vi "仪器参数发送 (子VI).vi"(8 "错误输入":errorcluster caption="错误输出") -> (0 "错误输出":errorcluster)   [LabVIEW 2016, in "数据传输系统.lvlib"]
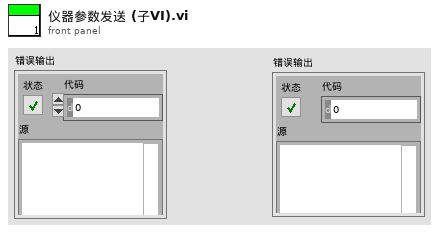
[diagram p1: front panel]
types:
  T1 = cluster{"氨氮仪器参数索引起始时间":string, "总磷仪器参数索引起始时间":string, "总氮仪器参数索引起始时间":string, "CODMn仪器参数索引起始时间":string, "CODCr仪器参数索引起始时间":string, "DO仪器参数索引起始时间":string, "PH仪器参数索引起始时间":string, "比电导率仪器参数索引起始时间":string, "水温仪器参数索引起始时间":string, "浊度仪器参数索引起始时间":string, "叶绿素a仪器参数索引起始时间":string, "藻密度仪器参数索引起始时间":string, "ORP仪器参数索引起始时间":string}
  T2 = cluster{"[0]":string, "[1]":string, "[2]":string, "[3]":string, "[4]":string, "[5]":string, "[6]":string, "[7]":string, "[8]":string, "[9]":string, "[10]":string, "[11]":string, "[12]":string}
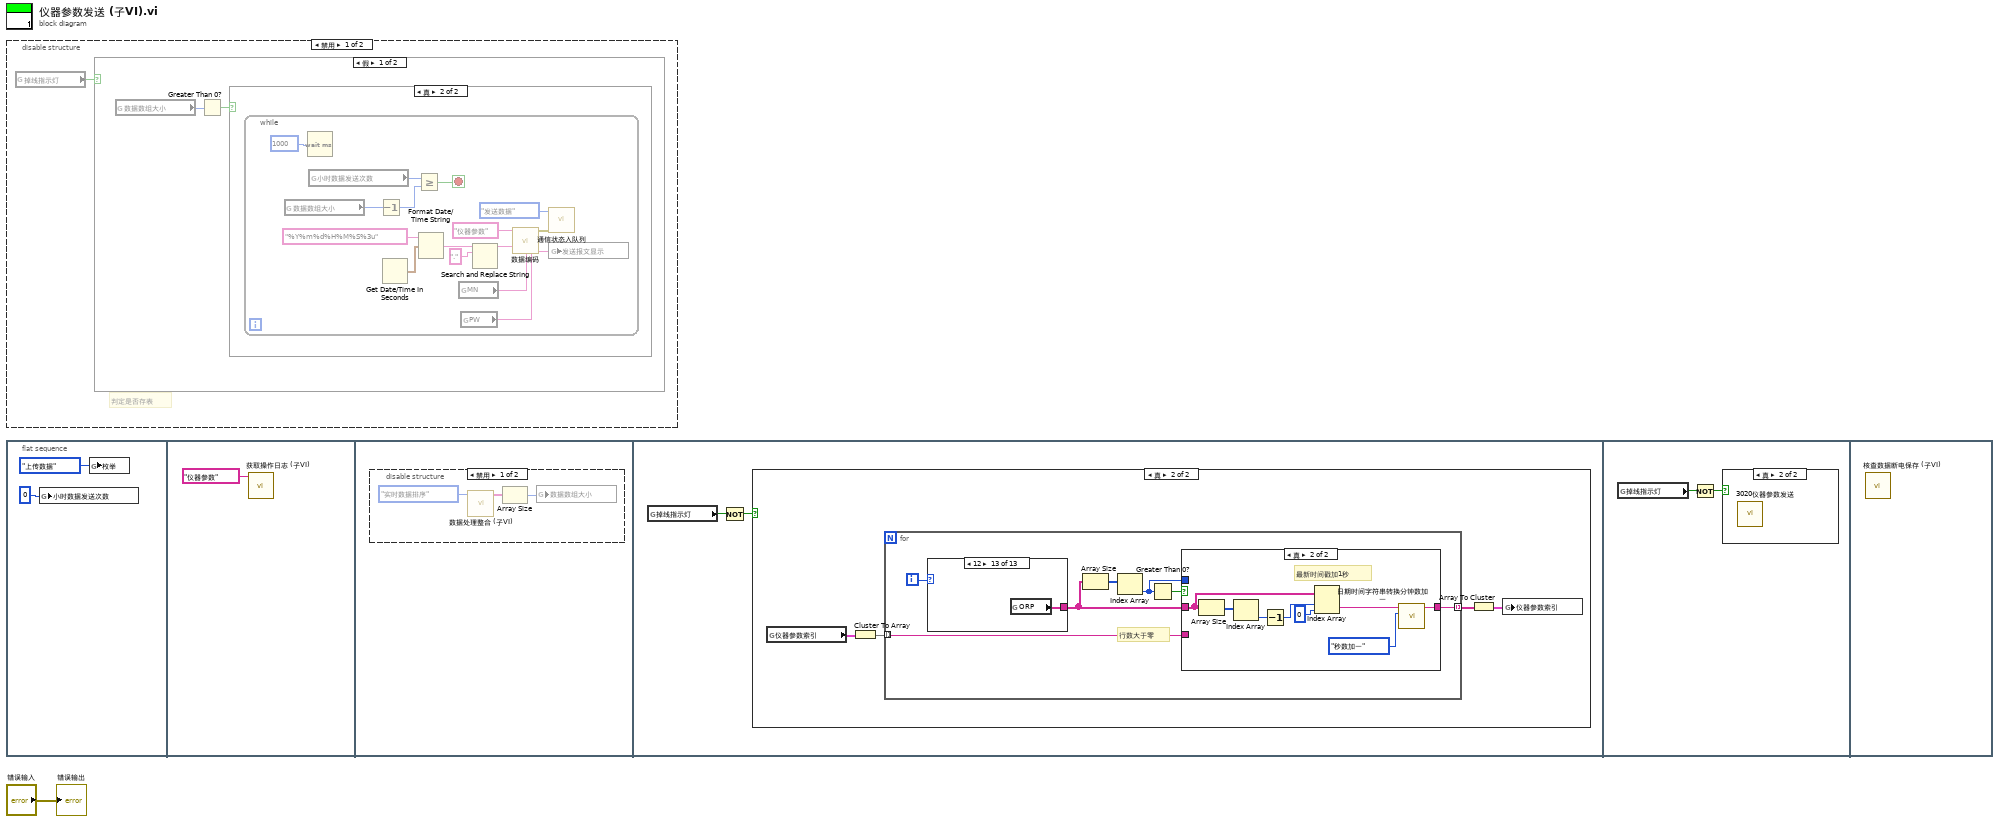
[diagram p0: block diagram]
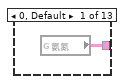
[diagram p7: hidden frame]
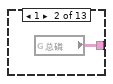
[diagram p8: hidden frame]
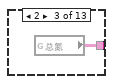
[diagram p9: hidden frame]
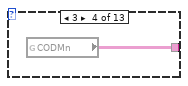
[diagram p10: hidden frame]
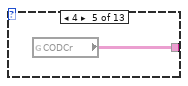
[diagram p11: hidden frame]
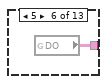
[diagram p12: hidden frame]
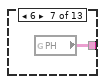
[diagram p13: hidden frame]
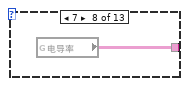
[diagram p14: hidden frame]
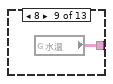
[diagram p15: hidden frame]
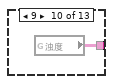
[diagram p16: hidden frame]
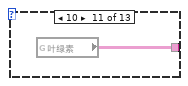
[diagram p17: hidden frame]
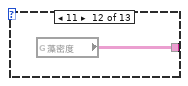
[diagram p18: hidden frame]
diagram:
  n1 = disable-structure shown="禁用" {
    frame Disabled {
      # "判定是否存表"
      n2 = global read "全局 数据发送重叠.vi" "掉线指示灯"() -> (w2:bool)
      n3 = case shown="假" w2 {
        frame False {
          n4 = global read "全局 数据数组大小.vi" "数据数组大小"() -> (w3:i32)
          n5 = Greater Than 0?(x=w3) -> (x > 0?=w4:bool)
          n6 = case shown="真" w4 {
            frame False {
            }
            frame True {
              n7 = while {
                stop <- w5 stop-if-true
                n8 = global read "全局 数据数组大小.vi" "数据数组大小"() -> (w7:i32)
                n9 = Wait (ms)(milliseconds to wait=u32 1000 ("等待时间（毫秒）")) -> ()  [unwired: 1 out]
                n10 = global read "全局 小时数据发送次数.vi" "小时数据发送次数"() -> (w8:i32)
                n11 = Decrement(x=w7) -> (x-1=w6:i32)
                n12 = Get Date/Time In Seconds() -> (seconds since 1Jan1904=w18:timestamp)
                n13 = Greater Or Equal?(x=w8, y=w6) -> (x >= y?=w5:bool)
                n14 = Format Date/Time String(time format string (%c)="%Y%m%d%H%M%S%3u" ("时间格式字符串(%c)"), seconds (now)=w18) -> (date/time string=w17:string)  [unwired: 1 in]
                n15 = global read "断电保存全局.vi" "MN"() -> (w12:string)
                n16 = global read "断电保存全局.vi" "PW"() -> (w11:string)
                n17 = Search and Replace String(input string=w17, search string="." ("搜索字符串")) -> (result string=w15:string)  [unwired: 6 in, 3 out]
                n18 = call "数据编码.vi"("table输入"="仪器参数" ("新元素/子数组"), "QN"=w15, "MN"=w12, "PW"=w11) -> ("错误常量"=w10:errorcluster, "通讯包字符串"=w14:string)  [unwired: 10 in]
                n19 = call "通信状态入队列.vi"("错误输入（无错误）"=w10, "枚举"=enum16{"打开连接", "发送数据", "读取数据", "数据处理", "关闭连接"}."发送数据") -> ()  [unwired: 9 in, 1 out]
                n20 = global write "全局1.vi" "发送报文显示"(w14) -> ()
              }
            }
          }
        }
        frame True {
        }
      }
    }
    frame Enabled {
    }
  }
  n21 = flat-sequence {
    frame #0 {
      n22 = global write "全局 小时数据发送次数.vi" "小时数据发送次数"(0 ("小时数据发送次数")) -> ()
      n23 = global write "全局1.vi" "枚举"(enum16{"返回请求应答", "上传数据", "返回执行结果"}."上传数据" ("枚举")) -> ()
    }
    frame #1 {
      n24 = call "获取操作日志 (子VI).vi"("table输入"="仪器参数") -> ()  [unwired: 11 in]
    }
    frame #2 {
      n25 = disable-structure shown="禁用" {
        frame Disabled {
          n26 = call "数据处理整合 (子VI).vi"("枚举"=enum16{"实时数据排序", "小时数据排序"}."实时数据排序") -> ("已排序的数组"=w26:string[])  [unwired: 10 in]
          n27 = Array Size(array=w26) -> (size(s)=w25:i32)
          n28 = global write "全局 数据数组大小.vi" "数据数组大小"(w25) -> ()
        }
        frame Enabled {
        }
      }
    }
    frame #3 {
      n29 = global read "全局 数据发送重叠.vi" "掉线指示灯"() -> (w28:bool)
      n30 = Not(x=w28) -> (.not. x?=w27:bool)
      n31 = case shown="真" w27 {
        frame False {
        }
        frame True {
          n32 = global read "全局 时间2.vi" "仪器参数索引"() -> (w32:T1)
          n33 = Cluster To Array(cluster=w32) -> (array=w31:string[])
          n34 = for {
            tunnel: [w36] -> w29 mode=indexing
            tunnel: w31 -> [w35] mode=indexing
            i -> [w34]
            # "行数大于零"
            n35 = case shown="12" w34 {
              tunnel: [w40 w41 w42 w43 w44 w45 w46 w47 w48 w49 w50 w51 w52] -> w33
              frame 0, Default {
                n36 = global read "全局 所有参数.vi" "氨氮"() -> (w40:string[][])
              }
              frame 1 {
                n37 = global read "全局 所有参数.vi" "总磷"() -> (w41:string[][])
              }
              frame 2 {
                n38 = global read "全局 所有参数.vi" "总氮"() -> (w42:string[][])
              }
              frame 3 {
                n39 = global read "全局 所有参数.vi" "CODMn"() -> (w43:string[][])
              }
              frame 4 {
                n40 = global read "全局 所有参数.vi" "CODCr"() -> (w44:string[][])
              }
              frame 5 {
                n41 = global read "全局 所有参数.vi" "DO"() -> (w45:string[][])
              }
              frame 6 {
                n42 = global read "全局 所有参数.vi" "PH"() -> (w46:string[][])
              }
              frame 7 {
                n43 = global read "全局 所有参数.vi" "电导率"() -> (w47:string[][])
              }
              frame 8 {
                n44 = global read "全局 所有参数.vi" "水温"() -> (w48:string[][])
              }
              frame 9 {
                n45 = global read "全局 所有参数.vi" "浊度"() -> (w49:string[][])
              }
              frame 10 {
                n46 = global read "全局 所有参数.vi" "叶绿素"() -> (w50:string[][])
              }
              frame 11 {
                n47 = global read "全局 所有参数.vi" "藻密度"() -> (w51:string[][])
              }
              frame 12 {
                n48 = global read "全局 所有参数.vi" "ORP"() -> (w52:string[][])
              }
            }
            n49 = Array Size(array=w33) -> (size(s)=w38:i32[])
            n50 = Index Array(array=w38) -> (element=w37:i32)  [unwired: 1 in]
            n51 = Greater Than 0?(x=w37) -> (x > 0?=w39:bool)
            n52 = case shown="真" w39 {
              tunnel: w37 -> [_ _]
              tunnel: w33 -> [_ w58]
              tunnel: [w53 w55] -> w36
              tunnel: w35 -> [w53 _]
              frame False {
              }
              frame True {
                # "最新时间戳加1秒"
                n53 = Array Size(array=w58) -> (size(s)=w60:i32[])
                n54 = Index Array(array=w60) -> (element=w59:i32)  [unwired: 1 in]
                n55 = Decrement(x=w59) -> (x-1=w57:i32)
                n56 = Index Array(array=w58, index (row)=w57, index (col)=0 ("禁用的索引 (列)")) -> (element=w61:string)
                n57 = call "日期时间字符串转换分钟数加一.vi"("枚举"=enum16{"分钟数加一", "秒数加一", "小时数加一"}."秒数加一", "data[0]"=w61) -> ("日期/时间字符串"=w55:string)  [unwired: 9 in]
              }
            }
          }
          n58 = Array To Cluster(array=w29) -> (cluster=w30:T2)
          n59 = global write "全局 时间2.vi" "仪器参数索引"(w30) -> ()
        }
      }
    }
    frame #4 {
      n60 = global read "全局 数据发送重叠.vi" "掉线指示灯"() -> (w63:bool)
      n61 = Not(x=w63) -> (.not. x?=w62:bool)
      n62 = case shown="真" w62 {
        frame False {
        }
        frame True {
          n63 = call "3020仪器参数发送.vi"() -> ()  [unwired: 12 in]
        }
      }
    }
    frame #5 {
      n64 = call "核查数据断电保存 (子VI).vi"() -> ()  [unwired: 12 in]
    }
  }
  "错误输出" <- "错误输入"
